vi "Toggle Hover.vi"(8 "error in (no error)":errorcluster, 10 "Index":i32, 11 "MCListbox with Checkboxes in":refnum<class "MCListbox with Checkboxes.lvclass">) -> (0 "error out":errorcluster, 3 "MCListbox with Checkboxes out":refnum<class "MCListbox with Checkboxes.lvclass">)   [LabVIEW 2016, in "MCListbox with Checkboxes.lvclass"]
uses:
  MCListbox with Checkboxes.lvclass
  MCListbox with Checkboxes.lvclass/MCListbox with Checkboxes.ctl
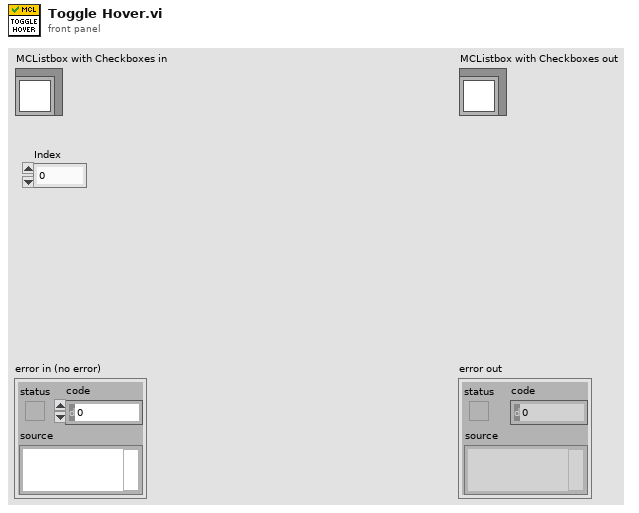
[diagram p1: front panel]
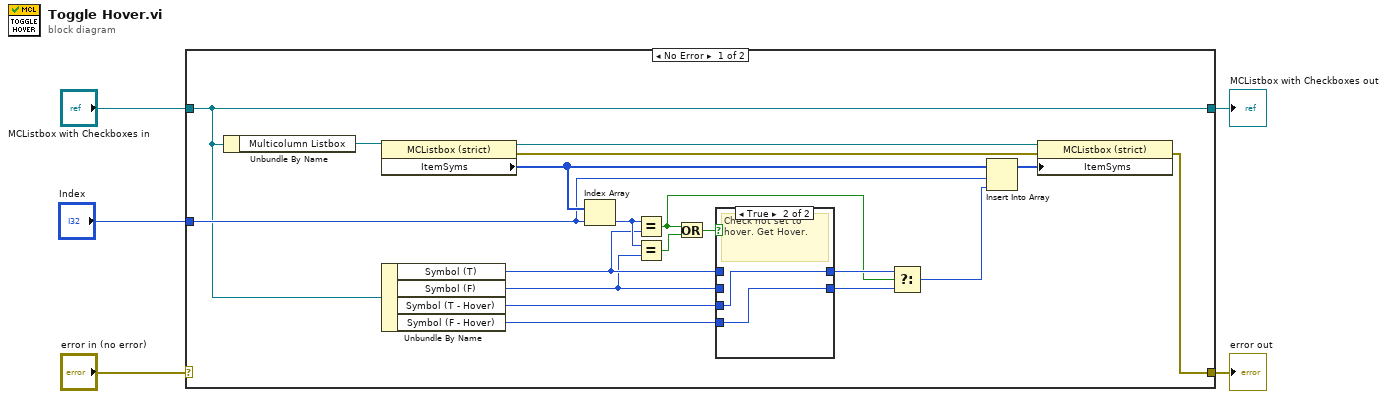
[diagram p0: block diagram]
diagram:
  n1 = case shown="No Error" "error in (no error)" {
    selector: "error in (no error)" -> [_ w30]
    tunnel: [w6 w30] -> w4
    tunnel: [w18 w29] -> w2
    tunnel: "MCListbox with Checkboxes in" -> [w18 w29]
    tunnel: "Index" -> [w19 _]
    frame No Error {
      n2 = Unbundle By Name(w18) -> ("Multicolumn Listbox"=w24:refnum<vi>)
      n3 = property class="MCListbox (strict)"(reference=w24) -> (reference out=w23:refnum<vi>, error out=w22:errorcluster, "ItemSyms"=w21:i32[])  [unwired: 1 in]
      n4 = Unbundle By Name(w18) -> ("Symbol (T)"=w12:i32, "Symbol (F)"=w11:i32, "Symbol (T - Hover)"=w14:i32, "Symbol (F - Hover)"=w13:i32)
      n5 = Index Array(array=w21, index=w19) -> (element=w17:i32)
      n6 = Equal?(x=w17, y=w12) -> (x = y?=w8:bool)
      n7 = Equal?(x=w17, y=w11) -> (x = y?=w16:bool)
      n8 = Or(x=w8, y=w16) -> (x .or. y?=w15:bool)
      n9 = case shown="True" w15 {
        tunnel: w14 -> [_ w28]
        tunnel: w13 -> [_ w27]
        tunnel: w12 -> [w26 _]
        tunnel: w11 -> [w25 _]
        tunnel: [w26 w28] -> w10
        tunnel: [w25 w27] -> w9
        frame False {
          # "Check set to hover. Get Basic."
        }
        frame True {
          # "Check not set to hover. Get Hover."
        }
      }
      n10 = Select(t=w10, s=w8, f=w9) -> (s? t:f=w7:i32)
      n11 = Insert Into Array(array=w21, index=w19, new element=w7) -> (w20:i32[])
      n12 = property class="MCListbox (strict)"(reference=w23, error in=w22, "ItemSyms"=w20) -> (error out=w6:errorcluster)  [unwired: 1 out]
    }
    frame Error {
    }
  }
  "error out" <- w4
  "MCListbox with Checkboxes out" <- w2
